vi "ProcessDifferentiation.vi"(8 "error in (no error)":errorcluster, 9 "parent waveform":waveform(sgl), 10 "parent found":bool, 11 "virtual channel":T1) -> (0 "error out":errorcluster, 2 "differentiated channel":waveform(sgl), 3 "virtual channel out":T1)   [LabVIEW 2017, in "CmsVirtualChannel.lvlib"]
uses:
  <vilib>/addons/InsightCM/Devices/Shared/Cms/CmsVirtualChannel/CmsVirtualChannel.lvlib
  <vilib>/addons/InsightCM/Devices/Shared/Cms/CmsVirtualChannel/controls/VirtualChannel.ctl
  <vilib>/addons/InsightCM/Devices/Shared/Cms/CmsVirtualChannel/controls/Differentiation.ctl
  <vilib>/addons/InsightCM/Utilities/Analysis/Shared/controls/ConversionOp.ctl
  <vilib>/addons/InsightCM/Utilities/Analysis/Shared/AnalysisHelper.lvlib
  <vilib>/addons/InsightCM/Utilities/ChannelStatus/ChannelStatus.lvlib
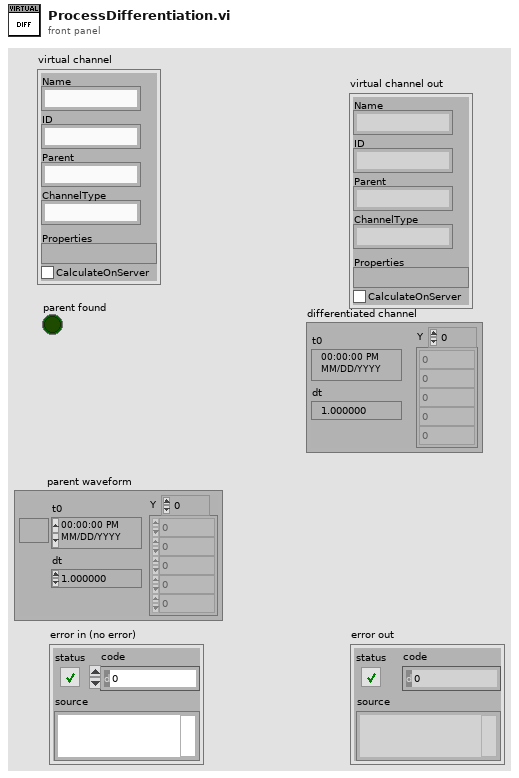
[diagram p1: front panel]
types:
  T1 = typedef "CmsVirtualChannel.lvlib/VirtualChannel.ctl" = cluster{"Name":string, "ID":string, "Parent":string, "ChannelType":string, "Properties":variant, "CalculateOnServer":bool}
  T2 = typedef "CmsVirtualChannel.lvlib/Differentiation.ctl" = cluster{"Conversion Op":T3, "Unit":string, "Parent Unit":string}
  T3 = typedef "AnalysisHelper.lvlib/ConversionOp.ctl" = enum16{"none", "singleInt", "doubleInt", "singleDiff", "doubleDiff"}
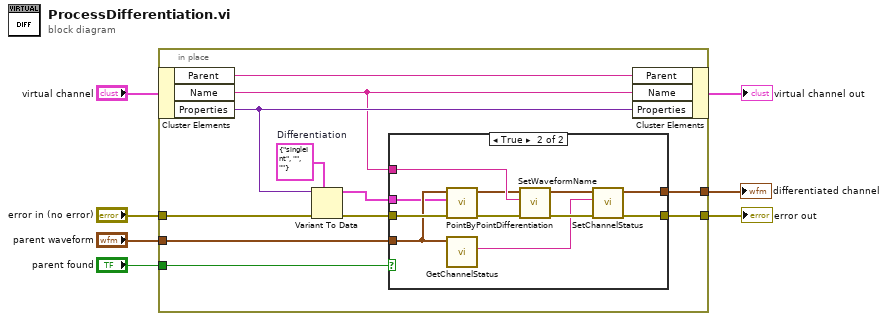
[diagram p0: block diagram]
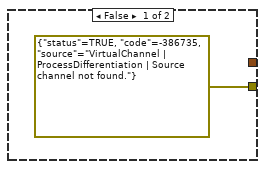
[diagram p2: hidden frame]
diagram:
  n1 = in-place {
    in-place-border: "error in (no error)" -> [w16]
    in-place-border: [w17] -> w4
    in-place-border: [w10] -> w3
    in-place-border: "parent found" -> [w9]
    in-place-border: "parent waveform" -> [w8]
    w13 = T2 {"Conversion Op"=enum."singleInt", "Unit"="", "Parent Unit"=""}  # Differentiation
    n2 = in-place-cluster #1("virtual channel") -> ("Parent"=w18:string, "Name"=w11:string, "Properties"=w12:variant)
    n3 = Variant To Data(error in=w16, type=w13, Variant=w12) -> (data=w14:T2, error out=w15:errorcluster)
    n4 = case shown="True" w9 {
      tunnel: w15 -> [_ w30]
      tunnel: [errorcluster {"status"=TRUE, "code"=-386735, "source"="VirtualChannel | ProcessDifferentiation | Source channel not found."} ("error in (no error)") w27] -> w17
      tunnel: w8 -> [_ w21]
      tunnel: w11 -> [_ w24]
      tunnel: w14 -> [_ w20]
      tunnel: [_ w28] -> w10
      frame False {
      }
      frame True {
        n5 = call <vilib>:"PointByPointDifferentiation.vi"("error in (no error)"=w30, "Differentiation"=w20, "Waveform"=w21) -> ("error out"=w29:errorcluster, "Differentiated Waveform"=w22:waveform(sgl))  [unwired: 7 in]
        n6 = call <vilib>:"GetChannelStatus.vi"("waveform in"=w21) -> ("channel status"=w25:string)  [unwired: 7 in, 3 out]
        n7 = call <vilib>:"SetWaveformName.vi"("error in (no error)"=w29, "Name"=w24, "Waveform in"=w22) -> ("error out"=w26:errorcluster, "Waveform out"=w23:waveform(sgl))  [unwired: 7 in]
        n8 = call <vilib>:"SetChannelStatus.vi"("error in (no error)"=w26, "Channel Status"=w25, "Waveform in"=w23) -> ("error out"=w27:errorcluster, "Waveform out"=w28:waveform(sgl))  [unwired: 7 in]
      }
    }
    n9 = in-place-cluster #1("Parent"=w18, "Name"=w11, "Properties"=w12) -> (→"virtual channel out":T1)
  }
  "error out" <- w4
  "differentiated channel" <- w3
